vi "ExtraLargeFileCompleteBroadcast_Send.vi"(8 "error in (no error)":errorcluster, 9 "data":variant, 11 "Qbus in":refnum<class "Qbus.lvclass">) -> (0 "error out":errorcluster)   [LabVIEW 2017, in "FileManager.lvlib"]
uses:
  <vilib>/addons/InsightCM/Devices/Shared/Common/FileManager/FileManager.lvlib
  <vilib>/addons/Qbus/Qbus.lvclass
  <vilib>/addons/InsightCM/Devices/Shared/Common/FileManager/controls/DataPropertyNames.ctl
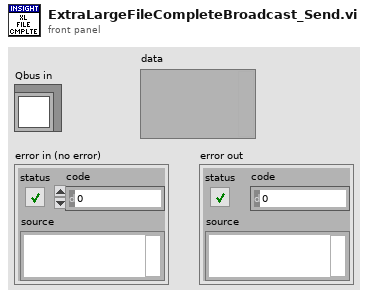
[diagram p1: front panel]
types:
  T1 = typedef "DataPropertyNames.ctl" = enum16{"Type", "EventRef", "FilePath", "DataGroup", "AcquisitionTimestamp", "StreamId", "StreamBlock", "TrendPointsOnly", "ExtraLargeFile"}
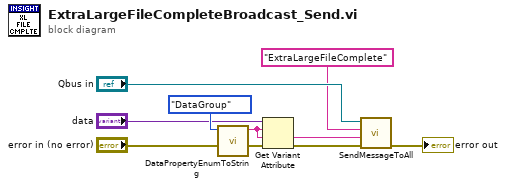
[diagram p0: block diagram]
diagram:
  n1 = call <vilib>:"DataPropertyEnumToString.vi"("property"=DataPropertyNames."DataGroup" ("Names")) -> ("string"=w4:string)  [unwired: 10 in]
  n2 = Get Variant Attribute(Variant="data", name=w4, default value (empty Variant)=w4, error in="error in (no error)") -> (value=w3:string, error out=w2:errorcluster)  [unwired: 2 out]
  n3 = call <vilib>:"SendMessageToAll.vi"("error in (no error)"=w2, "message value"=w3, "message name"="ExtraLargeFileComplete" ("MsgName"), "Qbus in"="Qbus in") -> ("error in (no error)"=→"error out":errorcluster)  [unwired: 6 in, 1 out]
